vi "tunel_contador.vi"() -> ()   [LabVIEW 2020]
panel:
  out "Numeric 4":dbl
  in  "stop":bool
  in  "Numeric":dbl
  out "Numeric 3":dbl
  in  "Numeric 2":dbl
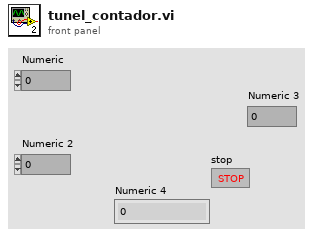
[diagram p1: front panel]
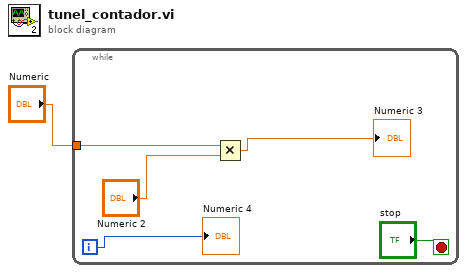
[diagram p0: block diagram]
diagram:
  n1 = while {
    tunnel: "Numeric" -> [w2]
    i -> [w3]
    stop <- "stop" stop-if-true
    n2 = Multiply(x=w2, y="Numeric 2") -> (x*y=→"Numeric 3":dbl)
    "Numeric 4" <- w3
  }
